vi "cameraControl.vi"(1 "Stream?":bool, 2 "Camera Parameters":T3 {"Pixel Format" items=["PIXEL_FORMAT_MONO8", "PIXEL_FORMAT_MONO16", "PIXEL_FORMAT_YUV422", "PIXEL_FORMAT_BAYER8_GRBG", "PIXEL_FORMAT_BAYER16_GRBG", "PIXEL_FORMAT_RGB24", "PIXEL_FORMAT_RGB48", "PIXEL_FORMAT_BAYER8_RGGB", "PIXEL_FORMAT_BAYER8_GBRG ", "PIXEL_FORMAT_BAYER8_BGGR ", "PIXEL_FORMAT_BAYER16_RGGB ", "PIXEL_FORMAT_BAYER16_GBRG", "PIXEL_FORMAT_BAYER16_BGGR", "PIXEL_FORMAT_RGB32"]}, 3 "Selector":u16(ring)) -> (0 "Camera Device OUT":T1)   [LabVIEW 2010]
uses:
  <vilib>/addons/PixeLINK/Low Level Functions/CAMERA_FEATURES.llb/TDPU-CameraFeatures-FeatureIds.ctl
  <vilib>/addons/PixeLINK/Low Level Functions/CAMERA_FEATURES.llb/TDPU-CameraFeatures-FeatureFlags.ctl
  <vilib>/addons/PixeLINK/Low Level Functions/CAMERA_FEATURES.llb/TDPU-CameraFeatures-PixelFormat.ctl
panel:
  in  "Camera Device IN":T1
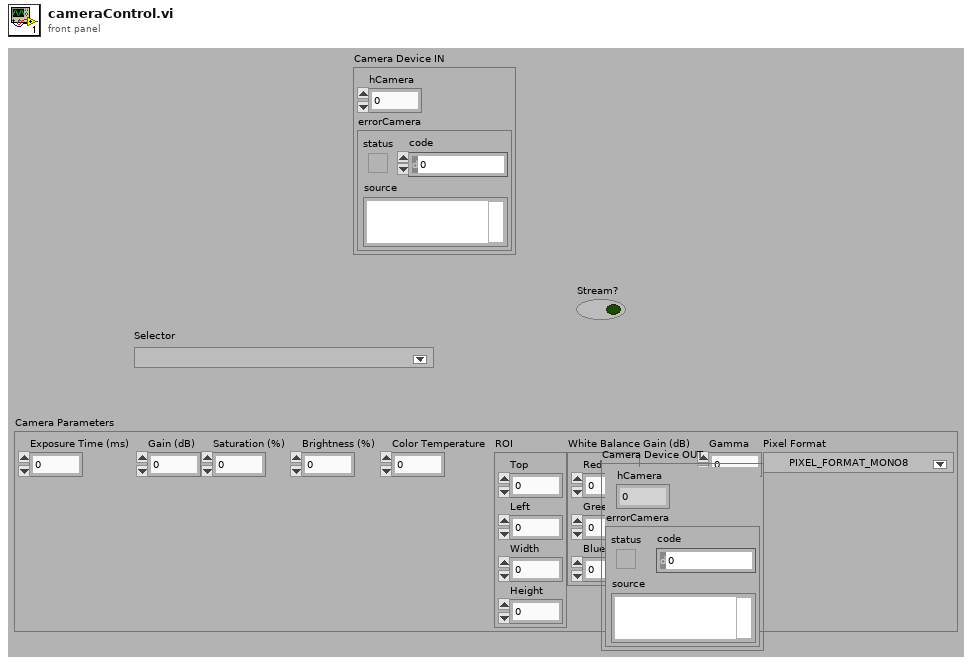
[diagram p1: front panel]
types:
  T1 = cluster{"hCamera":u32, "errorCamera":errorcluster}
  T2 = typedef "TDPU-CameraFeatures-PixelFormat.ctl" = u16
  T3 = cluster{"Exposure Time (ms)":dbl, "Gain (dB)":dbl, "Saturation (%)":dbl, "Brightness (%)":dbl, "Color Temperature":dbl, "ROI":cluster{"Top":i32, "Left":i32, "Width":i32, "Height":i32}, "White Balance Gain (dB)":cluster{"Red":dbl, "Green":dbl, "Blue":dbl}, "Gamma":dbl, "Pixel Format":T2}
  T4 = cluster{"Selector":u16, "Stream?":bool, "Camera Parameters":cluster{"Exposure Time (ms)":dbl, "Gain (dB)":dbl, "Saturation (%)":dbl, "Brightness (%)":dbl, "Color Temperature":dbl, "ROI":cluster{"Top":i32, "Left":i32, "Width":i32, "Height":i32}, "White Balance Gain (dB)":cluster{"Red":dbl, "Green":dbl, "Blue":dbl}, "Gamma":dbl, "Pixel Format":T2}}
  T5 = typedef "TDPU-CameraFeatures-FeatureFlags.ctl" = u32
  T6 = typedef "TDPU-CameraFeatures-FeatureIds.ctl" = u32
  T7 = cluster{"Top":i32, "Left":i32, "Width":i32, "Height":i32}
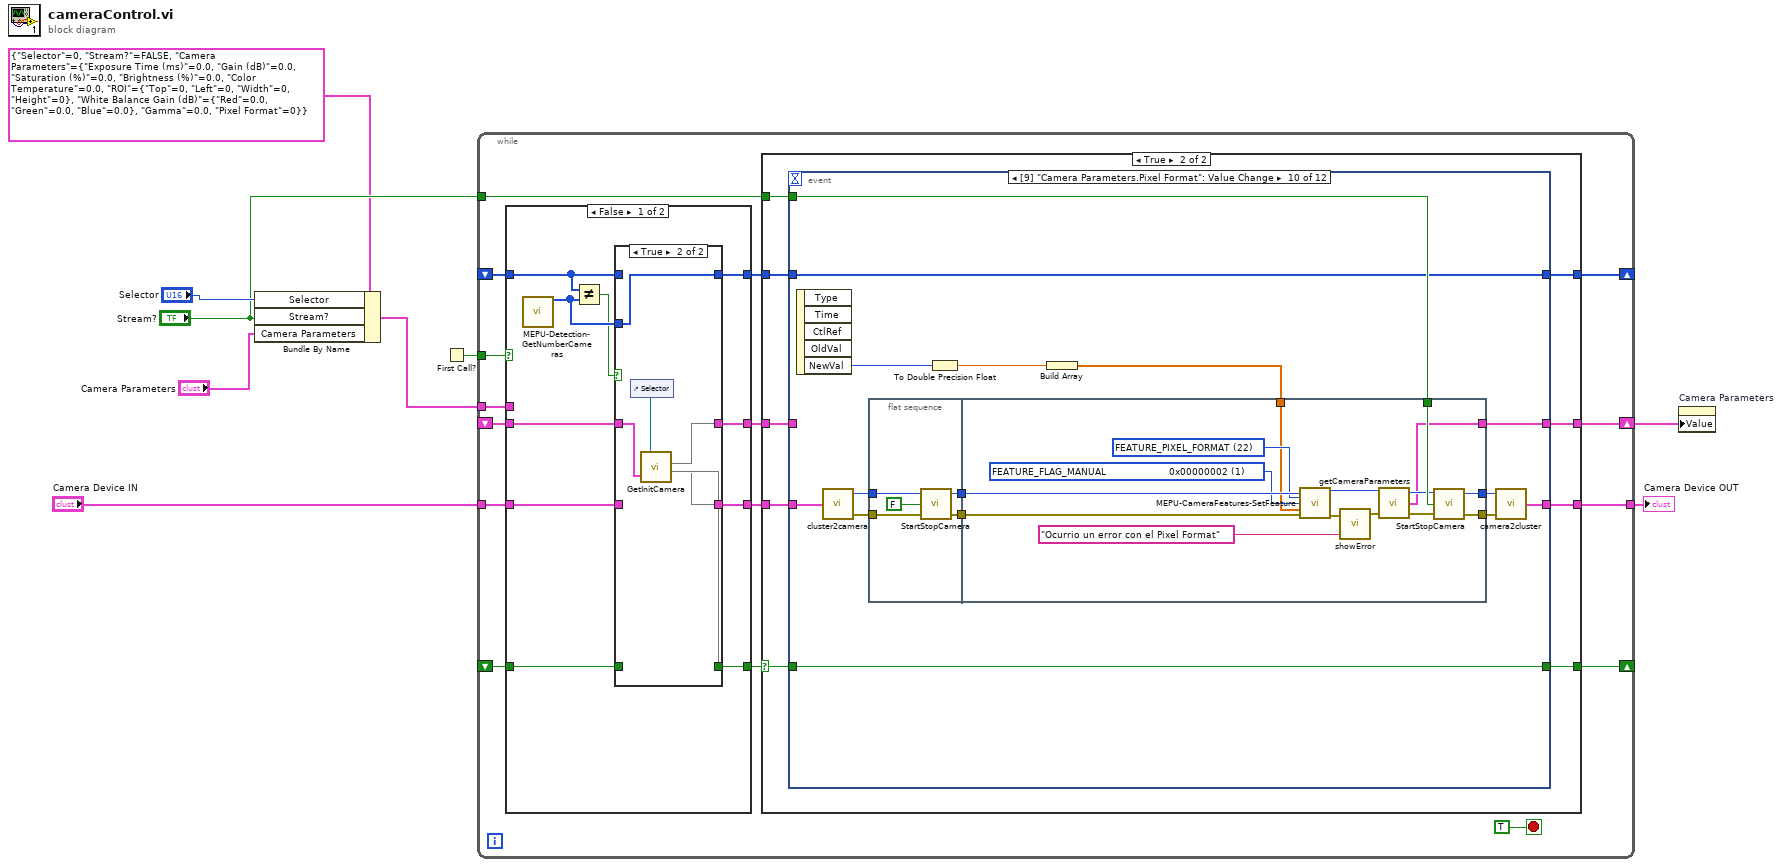
[diagram p0: block diagram]
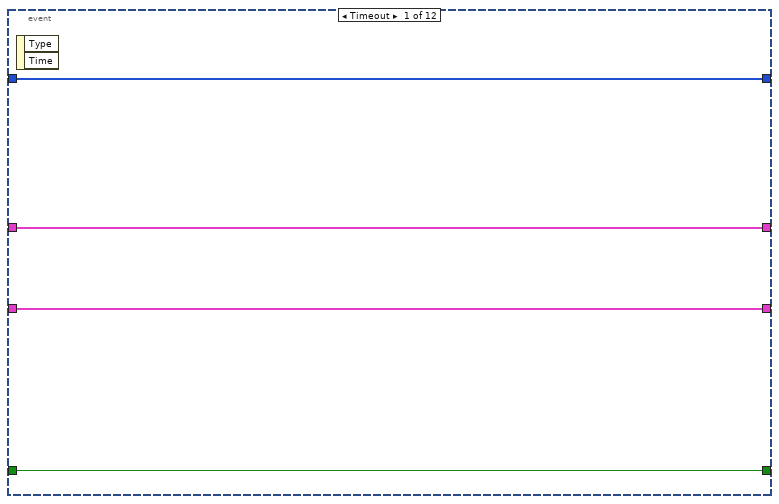
[diagram p3: hidden frame]
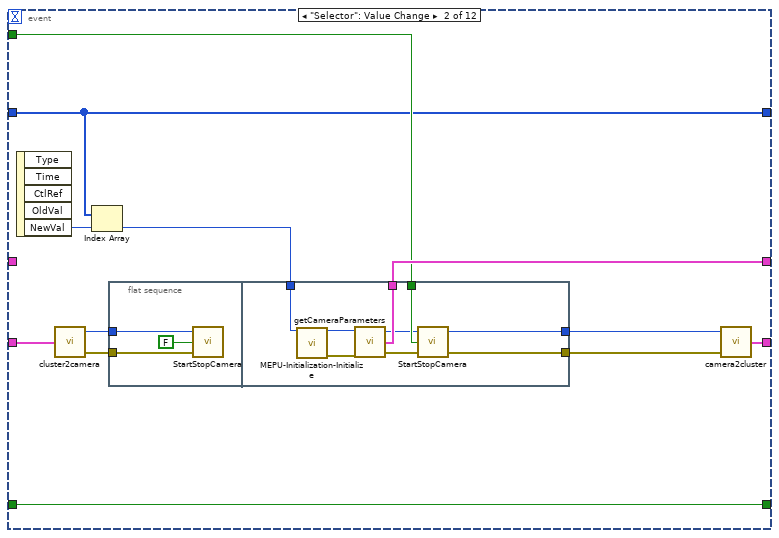
[diagram p4: hidden frame]
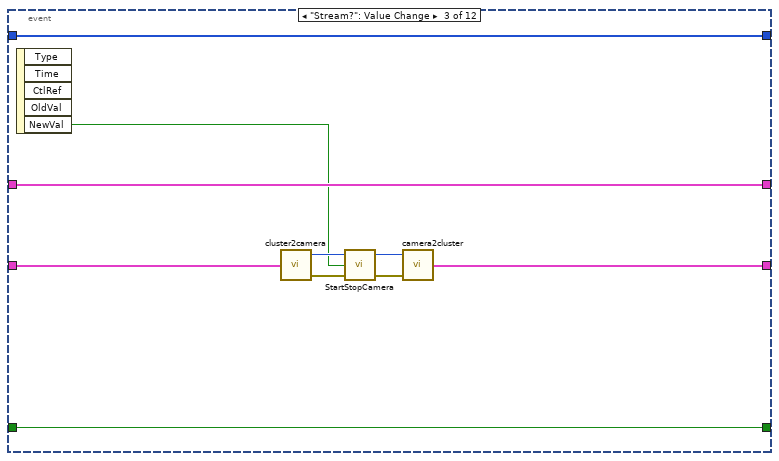
[diagram p5: hidden frame]
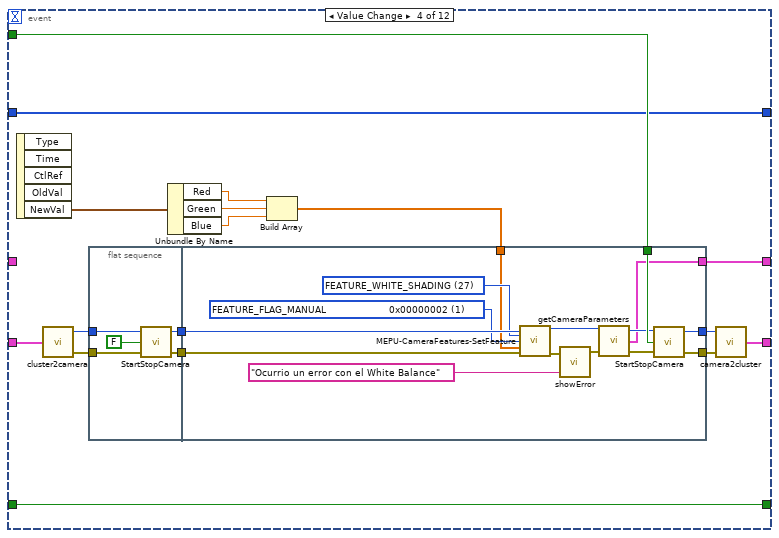
[diagram p6: hidden frame]
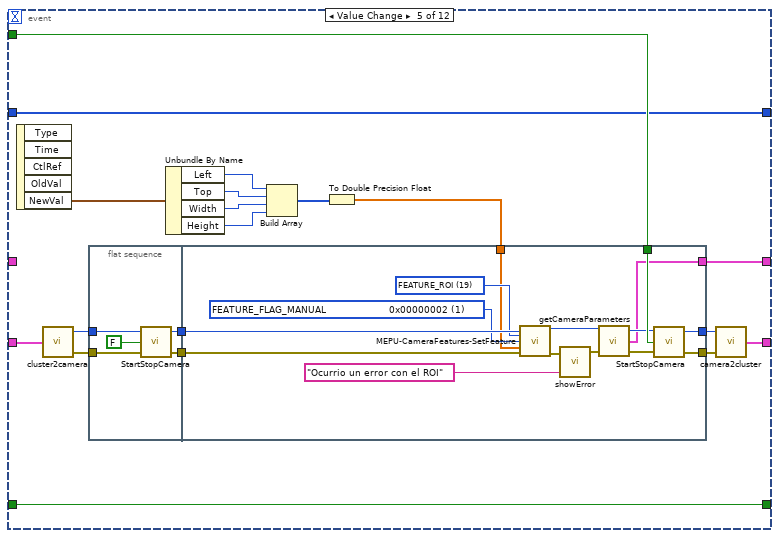
[diagram p7: hidden frame]
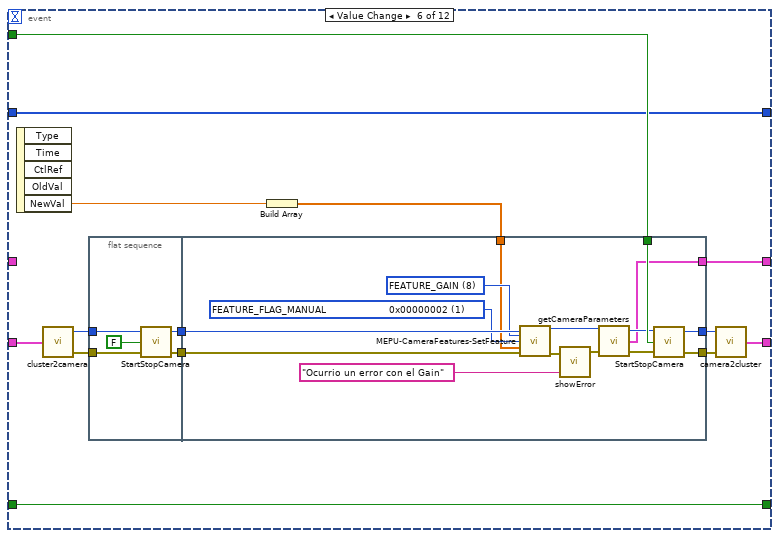
[diagram p8: hidden frame]
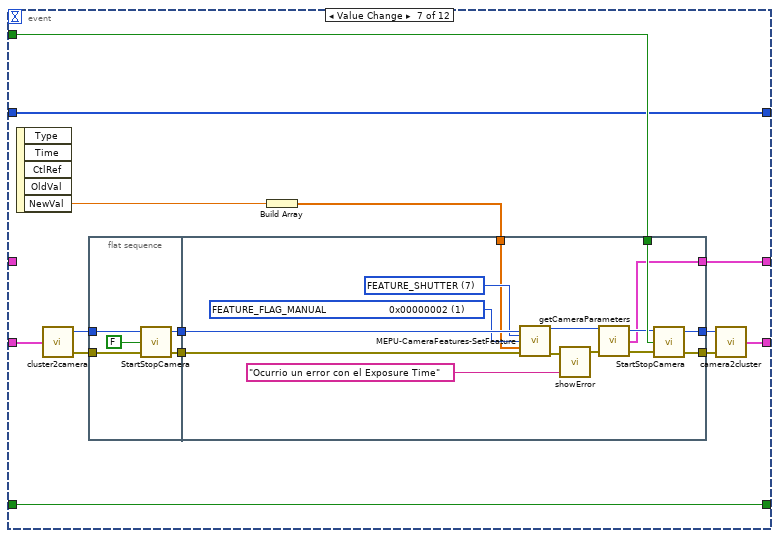
[diagram p9: hidden frame]
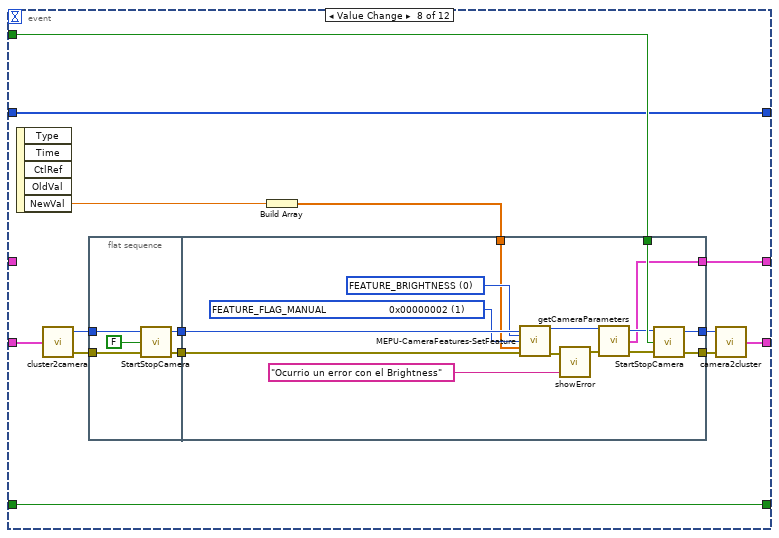
[diagram p10: hidden frame]
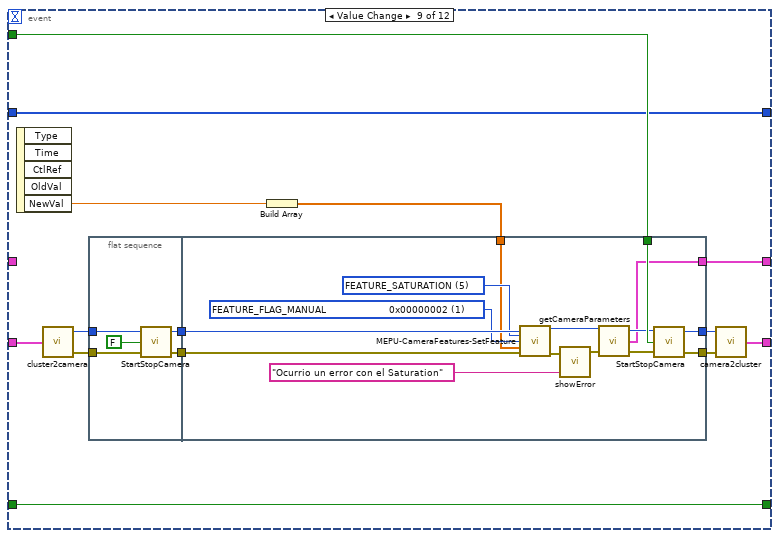
[diagram p11: hidden frame]
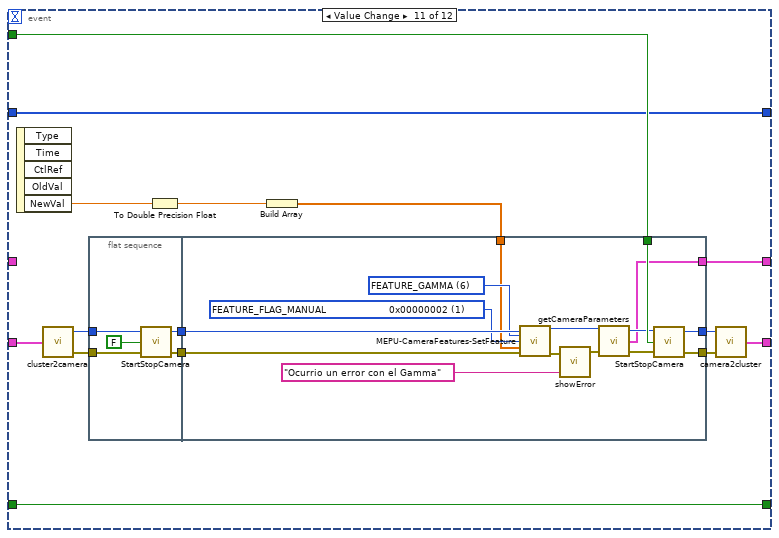
[diagram p12: hidden frame]
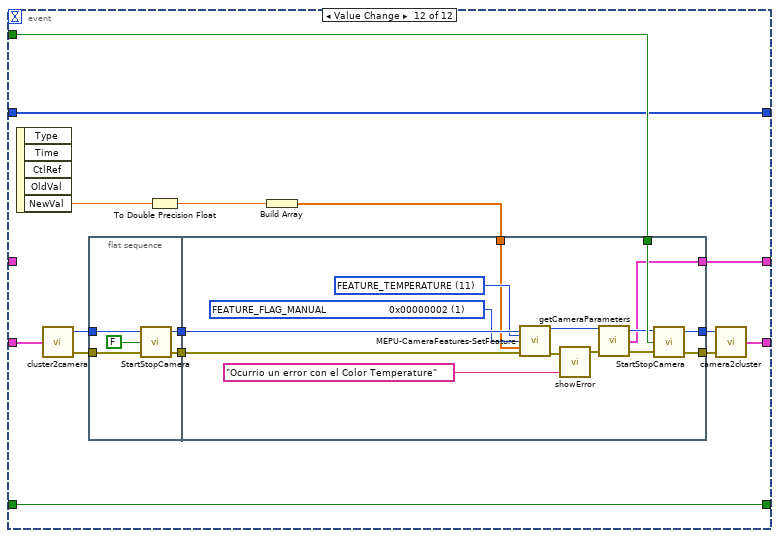
[diagram p13: hidden frame]
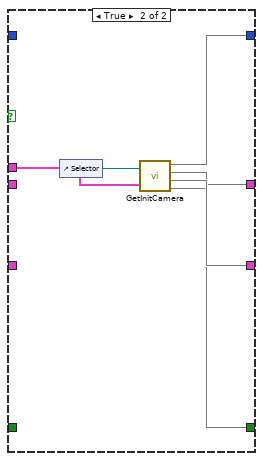
[diagram p15: hidden frame]
diagram:
  n1 = Bundle By Name(cluster=T4 {"Selector"=0, "Stream?"=FALSE, "Camera Parameters"={"Exposure Time (ms)"=0.0, "Gain (dB)"=0.0, "Saturation (%)"=0.0, "Brightness (%)"=0.0, "Color Temperature"=0.0, "ROI"={"Top"=0, "Left"=0, "Width"=0, "Height"=0}, "White Balance Gain (dB)"={"Red"=0.0, "Green"=0.0, "Blue"=0.0}, "Gamma"=0.0, "Pixel Format"=0}}, "Selector"="Selector", "Stream?"="Stream?", "Camera Parameters"="Camera Parameters") -> (w1:T4)
  n2 = First Call?() -> (First Call?: T/F=w9:bool)
  n3 = while {
    shift-right: [w23] -> w8
    shift-left: _ -> [w13]
    tunnel: "Stream?" -> [w22]
    tunnel: w9 -> [w19]
    shift-right: [w21] -> _
    shift-left: _ -> [w20]
    shift-right: [w18] -> _
    shift-left: _ -> [w12]
    tunnel: w1 -> [w11]
    tunnel: "Camera Device IN" -> [w15]
    tunnel: [w10] -> w7
    stop <- TRUE stop-if-true
    n4 = case shown="False" w19 {
      tunnel: [w400 w419] -> w24
      tunnel: w20 -> [w399 _]
      tunnel: [w402 w418] -> w17
      tunnel: [w403 w417] -> w16
      tunnel: w15 -> [w396 _]
      tunnel: [w401 w416] -> w14
      tunnel: w13 -> [w397 _]
      tunnel: w12 -> [w395 _]
      tunnel: w11 -> [_ w415]
      frame False {
        n5 = call <vilib>:"MEPU-Detection-GetNumberCameras.vi"() -> ("LV_SerialNumbers OUT"=w398:u32[])  [unwired: 13 in, 2 out]
        n6 = Not Equal?(x=w399, y=w398) -> (x != y?=w394:bool)
        n7 = case shown="True" w394 {
          tunnel: [w404 w413] -> w403
          tunnel: [w405 w412] -> w402
          tunnel: [w406 w411] -> w401
          tunnel: [w407 w408] -> w400
          tunnel: w399 -> [w407 _]
          tunnel: w398 -> [_ w408]
          tunnel: w397 -> [w406 w409]
          tunnel: w396 -> [w405 _]
          tunnel: w395 -> [w404 _]
          frame False {
          }
          frame True {
            n8 = control-ref of="Selector"() -> (w410:refnum<vi>)
            n9 = call "GetInitCamera.vi"(0:w409, 1:w410) -> (2:w413, 3:w412, 4:w411)  [unwired: 1 in]
          }
        }
      }
      frame True {
        n10 = control-ref of="Selector"() -> (w414:refnum<vi>)
        n11 = call "GetInitCamera.vi"(0:w415, 1:w414) -> (2:w417, 3:w418, 4:w416, 5:w419)
      }
    }
    n12 = case shown="True" w16 {
      selector: w16 -> [w26 w32]
      tunnel: w24 -> [w29 w38]
      tunnel: [w28 w37] -> w23
      tunnel: [w27 w36] -> w10
      tunnel: w22 -> [_ w35]
      tunnel: [w29 w34] -> w21
      tunnel: [w26 w33] -> w18
      tunnel: w17 -> [w27 w31]
      tunnel: w14 -> [w28 w30]
      frame False {
      }
      frame True {
        n13 = event shown="[9] \"Camera Parameters.Pixel Format\": Value Change" {
          selector: _ -> [_ _ _ _ _ _ _ _ _ _ _ _]
          dyn-events: _ -> [_ _ _ _ _ _ _ _ _ _ _ _]
          timeout: _ -> [_ _ _ _ _ _ _ _ _ _ _ _]
          tunnel: w38 -> [w40 w44 w69 w78 w117 w154 w188 w222 w256 w292 w327 w362]
          tunnel: [w42 w48 w70 w83 w122 w157 w191 w225 w259 w294 w329 w364] -> w37
          tunnel: [w41 w53 w75 w88 w127 w161 w195 w229 w263 w298 w333 w368] -> w36
          tunnel: w35 -> [_ w47 _ w85 w124 w158 w192 w226 w260 w295 w330 w365]
          tunnel: w30 -> [w42 _ w70 _ _ _ _ _ _ _ _ _]
          tunnel: w31 -> [w41 w52 w76 w89 w128 w162 w196 w230 w264 w299 w334 w369]
          tunnel: [w40 w44 w69 w78 w117 w154 w188 w222 w256 w292 w327 w362] -> w34
          tunnel: [w39 w43 w67 w77 w114 w153 w187 w221 w255 w289 w324 w359] -> w33
          tunnel: w32 -> [w39 w43 w67 w77 w114 w153 w187 w221 w255 w289 w324 w359]
          event Timeout {
            n14 = event-data() -> ()  [unwired: 1 in, 2 out]
          }
          event "Selector": Value Change {
            n15 = event-data() -> ("NewVal"=w54:u16)  [unwired: 1 in, 4 out]
            n16 = call "cluster2camera.vi"("Camera Device IN"=w52) -> ("Error OUT"=w50:errorcluster, "hCamera OUT"=w51:u32)  [unwired: 1 in]
            n17 = Index Array(array=w44, index=w54) -> (element=w49:u32)
            n18 = flat-sequence {
              tunnel: w51 -> [w56]
              tunnel: w50 -> [w55]
              tunnel: w49 -> [w66]
              tunnel: [w62] -> w48
              tunnel: w47 -> [w61]
              tunnel: [w59] -> w46
              tunnel: [w58] -> w45
              frame #0 {
                n19 = call "StartStopCamera.vi"("Error IN"=w55, "Camara ON?"=FALSE, "hCamera IN"=w56) -> ()  [unwired: 1 in, 2 out]
              }
              frame #1 {
                n20 = call <vilib>:"MEPU-Initialization-Initialize.vi"("uSerialNumber IN"=w66) -> ("phCamera OUT"=w65:u32, "Error OUT"=w64:errorcluster)  [unwired: 12 in, 1 out]
                n21 = call "getCameraParameters.vi"("Error IN"=w64, "hCamera IN"=w65) -> ("Error OUT"=w63:errorcluster, "Camera Parameters"=w62:T3, "hCamera OUT"=w60:u32)  [unwired: 1 in]
                n22 = call "StartStopCamera.vi"("Error IN"=w63, "Camara ON?"=w61, "hCamera IN"=w60) -> ("Error OUT"=w58:errorcluster, "hCamera OUT"=w59:u32)  [unwired: 1 in]
              }
            }
            n23 = call "camera2cluster.vi"("Error IN"=w45, "hCamera IN"=w46) -> ("Camera Device OUT"=w53:T1)  [unwired: 1 in]
          }
          event "Stream?": Value Change {
            n24 = event-data() -> ("NewVal"=w68:bool)  [unwired: 1 in, 4 out]
            n25 = call "cluster2camera.vi"("Camera Device IN"=w76) -> ("Error OUT"=w73:errorcluster, "hCamera OUT"=w74:u32)  [unwired: 1 in]
            n26 = call "StartStopCamera.vi"("Error IN"=w73, "Camara ON?"=w68, "hCamera IN"=w74) -> ("Error OUT"=w71:errorcluster, "hCamera OUT"=w72:u32)  [unwired: 1 in]
            n27 = call "camera2cluster.vi"("Error IN"=w71, "hCamera IN"=w72) -> ("Camera Device OUT"=w75:T1)  [unwired: 1 in]
          }
          event "Camera Parameters.White Balance Gain (dB)": Value Change {
            n28 = event-data() -> ("NewVal"=w84:cluster{"Red":dbl, "Green":dbl, "Blue":dbl})  [unwired: 1 in, 4 out]
            n29 = call "cluster2camera.vi"("Camera Device IN"=w89) -> ("Error OUT"=w92:errorcluster, "hCamera OUT"=w93:u32)  [unwired: 1 in]
            n30 = flat-sequence {
              tunnel: w93 -> [w97]
              tunnel: w92 -> [w96]
              tunnel: [w95] -> w87
              tunnel: [w94] -> w86
              tunnel: w85 -> [w113]
              tunnel: [w112] -> w91
              tunnel: [w111] -> w90
              tunnel: w87 -> [w110]
              tunnel: w86 -> [w109]
              tunnel: [w103] -> w83
              tunnel: w79 -> [w102]
              frame #0 {
                n31 = call "StartStopCamera.vi"("Error IN"=w96, "Camara ON?"=FALSE, "hCamera IN"=w97) -> ("Error OUT"=w94:errorcluster, "hCamera OUT"=w95:u32)  [unwired: 1 in]
              }
              frame #1 {
                w107 = T5 1 items=["FEATURE_FLAG_PRESENCE                 0x00000001", "FEATURE_FLAG_MANUAL                     0x00000002", "FEATURE_FLAG_AUTO                         0x00000004", "FEATURE_FLAG_ONEPUSH                   0x00000008", "FEATURE_FLAG_OFF                            0x00000010", "FEATURE_FLAG_DESC_SUPPORTED    0x00000020", "FEATURE_FLAG_READ_ONLY               0x00000040"] ("uFlags IN")
                w108 = T6 27 items=["FEATURE_BRIGHTNESS", "FEATURE_EXPOSURE", "FEATURE_SHARPNESS", "FEATURE_WHITE_BAL", "FEATURE_HUE", "FEATURE_SATURATION", "FEATURE_GAMMA", "FEATURE_SHUTTER", "FEATURE_GAIN", "FEATURE_IRIS", "FEATURE_FOCUS", "FEATURE_TEMPERATURE", "FEATURE_TRIGGER", "FEATURE_ZOOM", "FEATURE_PAN", "FEATURE_TILT", "FEATURE_OPT_FILTER", "FEATURE_GPIO", "FEATURE_FRAME_RATE", "FEATURE_ROI", "FEATURE_FLIP", "FEATURE_PIXEL_ADDRESSING", "FEATURE_PIXEL_FORMAT", "FEATURE_EXTENDED_SHUTTER", "FEATURE_AUTO_ROI", "FEATURE_LOOKUP_TABLE", "FEATURE_MEMORY_CHANNEL", "FEATURE_WHITE_SHADING", "FEATURE_ROTATE", "FEATURE_IMAGER_CLK_DIVISOR", "FEATURE_TRIG_WITH_CNTRLD_LIGHT", "FEATURE_MAX_PIXEL_SIZE"] ("uFeatureId IN")
                n32 = call <vilib>:"MEPU-CameraFeatures-SetFeature.vi"("hCamera IN"=w110, "uFeatureId IN"=w108, "uFlags IN"=w107, "pParms IN"=w102, "Error IN"=w109) -> ("hCamera OUT"=w106:u32, "Error OUT"=w101:errorcluster)  [unwired: 8 in, 1 out]
                n33 = call "showError.vi"("message"="Ocurrio un error con el White Balance", "Error IN"=w101) -> ("Error OUT"=w100:errorcluster)  [unwired: 3 in]
                n34 = call "getCameraParameters.vi"("Error IN"=w100, "hCamera IN"=w106) -> ("Error OUT"=w104:errorcluster, "Camera Parameters"=w103:T3, "hCamera OUT"=w105:u32)  [unwired: 1 in]
                n35 = call "StartStopCamera.vi"("Error IN"=w104, "Camara ON?"=w113, "hCamera IN"=w105) -> ("Error OUT"=w111:errorcluster, "hCamera OUT"=w112:u32)  [unwired: 1 in]
              }
            }
            n36 = Unbundle By Name(w84) -> ("Red"=w82:dbl, "Green"=w81:dbl, "Blue"=w80:dbl)
            n37 = Build Array(w82, w81, w80) -> (w79:dbl[])
            n38 = call "camera2cluster.vi"("Error IN"=w90, "hCamera IN"=w91) -> ("Camera Device OUT"=w88:T1)  [unwired: 1 in]
          }
          event "Camera Parameters.ROI": Value Change {
            n39 = event-data() -> ("NewVal"=w123:T7)  [unwired: 1 in, 4 out]
            n40 = call "cluster2camera.vi"("Camera Device IN"=w128) -> ("Error OUT"=w131:errorcluster, "hCamera OUT"=w132:u32)  [unwired: 1 in]
            n41 = flat-sequence {
              tunnel: w132 -> [w136]
              tunnel: w131 -> [w135]
              tunnel: [w134] -> w126
              tunnel: [w133] -> w125
              tunnel: w124 -> [w152]
              tunnel: [w151] -> w130
              tunnel: [w150] -> w129
              tunnel: w126 -> [w149]
              tunnel: w125 -> [w148]
              tunnel: [w142] -> w122
              tunnel: w115 -> [w141]
              frame #0 {
                n42 = call "StartStopCamera.vi"("Error IN"=w135, "Camara ON?"=FALSE, "hCamera IN"=w136) -> ("Error OUT"=w133:errorcluster, "hCamera OUT"=w134:u32)  [unwired: 1 in]
              }
              frame #1 {
                w146 = T5 1 items=["FEATURE_FLAG_PRESENCE                 0x00000001", "FEATURE_FLAG_MANUAL                     0x00000002", "FEATURE_FLAG_AUTO                         0x00000004", "FEATURE_FLAG_ONEPUSH                   0x00000008", "FEATURE_FLAG_OFF                            0x00000010", "FEATURE_FLAG_DESC_SUPPORTED    0x00000020", "FEATURE_FLAG_READ_ONLY               0x00000040"] ("uFlags IN")
                w147 = T6 19 items=["FEATURE_BRIGHTNESS", "FEATURE_EXPOSURE", "FEATURE_SHARPNESS", "FEATURE_WHITE_BAL", "FEATURE_HUE", "FEATURE_SATURATION", "FEATURE_GAMMA", "FEATURE_SHUTTER", "FEATURE_GAIN", "FEATURE_IRIS", "FEATURE_FOCUS", "FEATURE_TEMPERATURE", "FEATURE_TRIGGER", "FEATURE_ZOOM", "FEATURE_PAN", "FEATURE_TILT", "FEATURE_OPT_FILTER", "FEATURE_GPIO", "FEATURE_FRAME_RATE", "FEATURE_ROI", "FEATURE_FLIP", "FEATURE_PIXEL_ADDRESSING", "FEATURE_PIXEL_FORMAT", "FEATURE_EXTENDED_SHUTTER", "FEATURE_AUTO_ROI", "FEATURE_LOOKUP_TABLE", "FEATURE_MEMORY_CHANNEL", "FEATURE_WHITE_SHADING", "FEATURE_ROTATE", "FEATURE_IMAGER_CLK_DIVISOR", "FEATURE_TRIG_WITH_CNTRLD_LIGHT", "FEATURE_MAX_PIXEL_SIZE"] ("uFeatureId IN")
                n43 = call <vilib>:"MEPU-CameraFeatures-SetFeature.vi"("hCamera IN"=w149, "uFeatureId IN"=w147, "uFlags IN"=w146, "pParms IN"=w141, "Error IN"=w148) -> ("hCamera OUT"=w145:u32, "Error OUT"=w140:errorcluster)  [unwired: 8 in, 1 out]
                n44 = call "showError.vi"("message"="Ocurrio un error con el ROI", "Error IN"=w140) -> ("Error OUT"=w139:errorcluster)  [unwired: 3 in]
                n45 = call "getCameraParameters.vi"("Error IN"=w139, "hCamera IN"=w145) -> ("Error OUT"=w143:errorcluster, "Camera Parameters"=w142:T3, "hCamera OUT"=w144:u32)  [unwired: 1 in]
                n46 = call "StartStopCamera.vi"("Error IN"=w143, "Camara ON?"=w152, "hCamera IN"=w144) -> ("Error OUT"=w150:errorcluster, "hCamera OUT"=w151:u32)  [unwired: 1 in]
              }
            }
            n47 = Unbundle By Name(w123) -> ("Left"=w121:i32, "Top"=w120:i32, "Width"=w119:i32, "Height"=w118:i32)
            n48 = Build Array(w121, w120, w119, w118) -> (w116:i32[])
            n49 = To Double Precision Float(number=w116) -> (double precision float=w115:dbl[])
            n50 = call "camera2cluster.vi"("Error IN"=w129, "hCamera IN"=w130) -> ("Camera Device OUT"=w127:T1)  [unwired: 1 in]
          }
          event "Camera Parameters.Gain (dB)": Value Change {
            n51 = event-data() -> ("NewVal"=w155:dbl)  [unwired: 1 in, 4 out]
            n52 = call "cluster2camera.vi"("Camera Device IN"=w162) -> ("Error OUT"=w165:errorcluster, "hCamera OUT"=w166:u32)  [unwired: 1 in]
            n53 = flat-sequence {
              tunnel: w166 -> [w170]
              tunnel: w165 -> [w169]
              tunnel: [w168] -> w160
              tunnel: [w167] -> w159
              tunnel: w158 -> [w186]
              tunnel: [w185] -> w164
              tunnel: [w184] -> w163
              tunnel: w160 -> [w183]
              tunnel: w159 -> [w182]
              tunnel: [w176] -> w157
              tunnel: w156 -> [w175]
              frame #0 {
                n54 = call "StartStopCamera.vi"("Error IN"=w169, "Camara ON?"=FALSE, "hCamera IN"=w170) -> ("Error OUT"=w167:errorcluster, "hCamera OUT"=w168:u32)  [unwired: 1 in]
              }
              frame #1 {
                w180 = T5 1 items=["FEATURE_FLAG_PRESENCE                 0x00000001", "FEATURE_FLAG_MANUAL                     0x00000002", "FEATURE_FLAG_AUTO                         0x00000004", "FEATURE_FLAG_ONEPUSH                   0x00000008", "FEATURE_FLAG_OFF                            0x00000010", "FEATURE_FLAG_DESC_SUPPORTED    0x00000020", "FEATURE_FLAG_READ_ONLY               0x00000040"] ("uFlags IN")
                w181 = T6 8 items=["FEATURE_BRIGHTNESS", "FEATURE_EXPOSURE", "FEATURE_SHARPNESS", "FEATURE_WHITE_BAL", "FEATURE_HUE", "FEATURE_SATURATION", "FEATURE_GAMMA", "FEATURE_SHUTTER", "FEATURE_GAIN", "FEATURE_IRIS", "FEATURE_FOCUS", "FEATURE_TEMPERATURE", "FEATURE_TRIGGER", "FEATURE_ZOOM", "FEATURE_PAN", "FEATURE_TILT", "FEATURE_OPT_FILTER", "FEATURE_GPIO", "FEATURE_FRAME_RATE", "FEATURE_ROI", "FEATURE_FLIP", "FEATURE_PIXEL_ADDRESSING", "FEATURE_PIXEL_FORMAT", "FEATURE_EXTENDED_SHUTTER", "FEATURE_AUTO_ROI", "FEATURE_LOOKUP_TABLE", "FEATURE_MEMORY_CHANNEL", "FEATURE_WHITE_SHADING", "FEATURE_ROTATE", "FEATURE_IMAGER_CLK_DIVISOR", "FEATURE_TRIG_WITH_CNTRLD_LIGHT", "FEATURE_MAX_PIXEL_SIZE"] ("uFeatureId IN")
                n55 = call <vilib>:"MEPU-CameraFeatures-SetFeature.vi"("hCamera IN"=w183, "uFeatureId IN"=w181, "uFlags IN"=w180, "pParms IN"=w175, "Error IN"=w182) -> ("hCamera OUT"=w179:u32, "Error OUT"=w174:errorcluster)  [unwired: 8 in, 1 out]
                n56 = call "showError.vi"("message"="Ocurrio un error con el Gain", "Error IN"=w174) -> ("Error OUT"=w173:errorcluster)  [unwired: 3 in]
                n57 = call "getCameraParameters.vi"("Error IN"=w173, "hCamera IN"=w179) -> ("Error OUT"=w177:errorcluster, "Camera Parameters"=w176:T3, "hCamera OUT"=w178:u32)  [unwired: 1 in]
                n58 = call "StartStopCamera.vi"("Error IN"=w177, "Camara ON?"=w186, "hCamera IN"=w178) -> ("Error OUT"=w184:errorcluster, "hCamera OUT"=w185:u32)  [unwired: 1 in]
              }
            }
            n59 = Build Array(w155) -> (w156:dbl[])
            n60 = call "camera2cluster.vi"("Error IN"=w163, "hCamera IN"=w164) -> ("Camera Device OUT"=w161:T1)  [unwired: 1 in]
          }
          event "Camera Parameters.Exposure Time (ms)": Value Change {
            n61 = event-data() -> ("NewVal"=w189:dbl)  [unwired: 1 in, 4 out]
            n62 = call "cluster2camera.vi"("Camera Device IN"=w196) -> ("Error OUT"=w199:errorcluster, "hCamera OUT"=w200:u32)  [unwired: 1 in]
            n63 = flat-sequence {
              tunnel: w200 -> [w204]
              tunnel: w199 -> [w203]
              tunnel: [w202] -> w194
              tunnel: [w201] -> w193
              tunnel: w192 -> [w220]
              tunnel: [w219] -> w198
              tunnel: [w218] -> w197
              tunnel: w194 -> [w217]
              tunnel: w193 -> [w216]
              tunnel: [w210] -> w191
              tunnel: w190 -> [w209]
              frame #0 {
                n64 = call "StartStopCamera.vi"("Error IN"=w203, "Camara ON?"=FALSE, "hCamera IN"=w204) -> ("Error OUT"=w201:errorcluster, "hCamera OUT"=w202:u32)  [unwired: 1 in]
              }
              frame #1 {
                w214 = T5 1 items=["FEATURE_FLAG_PRESENCE                 0x00000001", "FEATURE_FLAG_MANUAL                     0x00000002", "FEATURE_FLAG_AUTO                         0x00000004", "FEATURE_FLAG_ONEPUSH                   0x00000008", "FEATURE_FLAG_OFF                            0x00000010", "FEATURE_FLAG_DESC_SUPPORTED    0x00000020", "FEATURE_FLAG_READ_ONLY               0x00000040"] ("uFlags IN")
                w215 = T6 7 items=["FEATURE_BRIGHTNESS", "FEATURE_EXPOSURE", "FEATURE_SHARPNESS", "FEATURE_WHITE_BAL", "FEATURE_HUE", "FEATURE_SATURATION", "FEATURE_GAMMA", "FEATURE_SHUTTER", "FEATURE_GAIN", "FEATURE_IRIS", "FEATURE_FOCUS", "FEATURE_TEMPERATURE", "FEATURE_TRIGGER", "FEATURE_ZOOM", "FEATURE_PAN", "FEATURE_TILT", "FEATURE_OPT_FILTER", "FEATURE_GPIO", "FEATURE_FRAME_RATE", "FEATURE_ROI", "FEATURE_FLIP", "FEATURE_PIXEL_ADDRESSING", "FEATURE_PIXEL_FORMAT", "FEATURE_EXTENDED_SHUTTER", "FEATURE_AUTO_ROI", "FEATURE_LOOKUP_TABLE", "FEATURE_MEMORY_CHANNEL", "FEATURE_WHITE_SHADING", "FEATURE_ROTATE", "FEATURE_IMAGER_CLK_DIVISOR", "FEATURE_TRIG_WITH_CNTRLD_LIGHT", "FEATURE_MAX_PIXEL_SIZE"] ("uFeatureId IN")
                n65 = call <vilib>:"MEPU-CameraFeatures-SetFeature.vi"("hCamera IN"=w217, "uFeatureId IN"=w215, "uFlags IN"=w214, "pParms IN"=w209, "Error IN"=w216) -> ("hCamera OUT"=w213:u32, "Error OUT"=w208:errorcluster)  [unwired: 8 in, 1 out]
                n66 = call "showError.vi"("message"="Ocurrio un error con el Exposure Time", "Error IN"=w208) -> ("Error OUT"=w207:errorcluster)  [unwired: 3 in]
                n67 = call "getCameraParameters.vi"("Error IN"=w207, "hCamera IN"=w213) -> ("Error OUT"=w211:errorcluster, "Camera Parameters"=w210:T3, "hCamera OUT"=w212:u32)  [unwired: 1 in]
                n68 = call "StartStopCamera.vi"("Error IN"=w211, "Camara ON?"=w220, "hCamera IN"=w212) -> ("Error OUT"=w218:errorcluster, "hCamera OUT"=w219:u32)  [unwired: 1 in]
              }
            }
            n69 = Build Array(w189) -> (w190:dbl[])
            n70 = call "camera2cluster.vi"("Error IN"=w197, "hCamera IN"=w198) -> ("Camera Device OUT"=w195:T1)  [unwired: 1 in]
          }
          event "Camera Parameters.Brightness (%)": Value Change {
            n71 = event-data() -> ("NewVal"=w223:dbl)  [unwired: 1 in, 4 out]
            n72 = call "cluster2camera.vi"("Camera Device IN"=w230) -> ("Error OUT"=w233:errorcluster, "hCamera OUT"=w234:u32)  [unwired: 1 in]
            n73 = flat-sequence {
              tunnel: w234 -> [w238]
              tunnel: w233 -> [w237]
              tunnel: [w236] -> w228
              tunnel: [w235] -> w227
              tunnel: w226 -> [w254]
              tunnel: [w253] -> w232
              tunnel: [w252] -> w231
              tunnel: w228 -> [w251]
              tunnel: w227 -> [w250]
              tunnel: [w244] -> w225
              tunnel: w224 -> [w243]
              frame #0 {
                n74 = call "StartStopCamera.vi"("Error IN"=w237, "Camara ON?"=FALSE, "hCamera IN"=w238) -> ("Error OUT"=w235:errorcluster, "hCamera OUT"=w236:u32)  [unwired: 1 in]
              }
              frame #1 {
                w248 = T5 1 items=["FEATURE_FLAG_PRESENCE                 0x00000001", "FEATURE_FLAG_MANUAL                     0x00000002", "FEATURE_FLAG_AUTO                         0x00000004", "FEATURE_FLAG_ONEPUSH                   0x00000008", "FEATURE_FLAG_OFF                            0x00000010", "FEATURE_FLAG_DESC_SUPPORTED    0x00000020", "FEATURE_FLAG_READ_ONLY               0x00000040"] ("uFlags IN")
                w249 = T6 0 items=["FEATURE_BRIGHTNESS", "FEATURE_EXPOSURE", "FEATURE_SHARPNESS", "FEATURE_WHITE_BAL", "FEATURE_HUE", "FEATURE_SATURATION", "FEATURE_GAMMA", "FEATURE_SHUTTER", "FEATURE_GAIN", "FEATURE_IRIS", "FEATURE_FOCUS", "FEATURE_TEMPERATURE", "FEATURE_TRIGGER", "FEATURE_ZOOM", "FEATURE_PAN", "FEATURE_TILT", "FEATURE_OPT_FILTER", "FEATURE_GPIO", "FEATURE_FRAME_RATE", "FEATURE_ROI", "FEATURE_FLIP", "FEATURE_PIXEL_ADDRESSING", "FEATURE_PIXEL_FORMAT", "FEATURE_EXTENDED_SHUTTER", "FEATURE_AUTO_ROI", "FEATURE_LOOKUP_TABLE", "FEATURE_MEMORY_CHANNEL", "FEATURE_WHITE_SHADING", "FEATURE_ROTATE", "FEATURE_IMAGER_CLK_DIVISOR", "FEATURE_TRIG_WITH_CNTRLD_LIGHT", "FEATURE_MAX_PIXEL_SIZE"] ("uFeatureId IN")
                n75 = call <vilib>:"MEPU-CameraFeatures-SetFeature.vi"("hCamera IN"=w251, "uFeatureId IN"=w249, "uFlags IN"=w248, "pParms IN"=w243, "Error IN"=w250) -> ("hCamera OUT"=w247:u32, "Error OUT"=w242:errorcluster)  [unwired: 8 in, 1 out]
                n76 = call "showError.vi"("message"="Ocurrio un error con el Brightness", "Error IN"=w242) -> ("Error OUT"=w241:errorcluster)  [unwired: 3 in]
                n77 = call "getCameraParameters.vi"("Error IN"=w241, "hCamera IN"=w247) -> ("Error OUT"=w245:errorcluster, "Camera Parameters"=w244:T3, "hCamera OUT"=w246:u32)  [unwired: 1 in]
                n78 = call "StartStopCamera.vi"("Error IN"=w245, "Camara ON?"=w254, "hCamera IN"=w246) -> ("Error OUT"=w252:errorcluster, "hCamera OUT"=w253:u32)  [unwired: 1 in]
              }
            }
            n79 = Build Array(w223) -> (w224:dbl[])
            n80 = call "camera2cluster.vi"("Error IN"=w231, "hCamera IN"=w232) -> ("Camera Device OUT"=w229:T1)  [unwired: 1 in]
          }
          event "Camera Parameters.Saturation (%)": Value Change {
            n81 = event-data() -> ("NewVal"=w257:dbl)  [unwired: 1 in, 4 out]
            n82 = call "cluster2camera.vi"("Camera Device IN"=w264) -> ("Error OUT"=w267:errorcluster, "hCamera OUT"=w268:u32)  [unwired: 1 in]
            n83 = flat-sequence {
              tunnel: w268 -> [w272]
              tunnel: w267 -> [w271]
              tunnel: [w270] -> w262
              tunnel: [w269] -> w261
              tunnel: w260 -> [w288]
              tunnel: [w287] -> w266
              tunnel: [w286] -> w265
              tunnel: w262 -> [w285]
              tunnel: w261 -> [w284]
              tunnel: [w278] -> w259
              tunnel: w258 -> [w277]
              frame #0 {
                n84 = call "StartStopCamera.vi"("Error IN"=w271, "Camara ON?"=FALSE, "hCamera IN"=w272) -> ("Error OUT"=w269:errorcluster, "hCamera OUT"=w270:u32)  [unwired: 1 in]
              }
              frame #1 {
                w282 = T5 1 items=["FEATURE_FLAG_PRESENCE                 0x00000001", "FEATURE_FLAG_MANUAL                     0x00000002", "FEATURE_FLAG_AUTO                         0x00000004", "FEATURE_FLAG_ONEPUSH                   0x00000008", "FEATURE_FLAG_OFF                            0x00000010", "FEATURE_FLAG_DESC_SUPPORTED    0x00000020", "FEATURE_FLAG_READ_ONLY               0x00000040"] ("uFlags IN")
                w283 = T6 5 items=["FEATURE_BRIGHTNESS", "FEATURE_EXPOSURE", "FEATURE_SHARPNESS", "FEATURE_WHITE_BAL", "FEATURE_HUE", "FEATURE_SATURATION", "FEATURE_GAMMA", "FEATURE_SHUTTER", "FEATURE_GAIN", "FEATURE_IRIS", "FEATURE_FOCUS", "FEATURE_TEMPERATURE", "FEATURE_TRIGGER", "FEATURE_ZOOM", "FEATURE_PAN", "FEATURE_TILT", "FEATURE_OPT_FILTER", "FEATURE_GPIO", "FEATURE_FRAME_RATE", "FEATURE_ROI", "FEATURE_FLIP", "FEATURE_PIXEL_ADDRESSING", "FEATURE_PIXEL_FORMAT", "FEATURE_EXTENDED_SHUTTER", "FEATURE_AUTO_ROI", "FEATURE_LOOKUP_TABLE", "FEATURE_MEMORY_CHANNEL", "FEATURE_WHITE_SHADING", "FEATURE_ROTATE", "FEATURE_IMAGER_CLK_DIVISOR", "FEATURE_TRIG_WITH_CNTRLD_LIGHT", "FEATURE_MAX_PIXEL_SIZE"] ("uFeatureId IN")
                n85 = call <vilib>:"MEPU-CameraFeatures-SetFeature.vi"("hCamera IN"=w285, "uFeatureId IN"=w283, "uFlags IN"=w282, "pParms IN"=w277, "Error IN"=w284) -> ("hCamera OUT"=w281:u32, "Error OUT"=w276:errorcluster)  [unwired: 8 in, 1 out]
                n86 = call "showError.vi"("message"="Ocurrio un error con el Saturation", "Error IN"=w276) -> ("Error OUT"=w275:errorcluster)  [unwired: 3 in]
                n87 = call "getCameraParameters.vi"("Error IN"=w275, "hCamera IN"=w281) -> ("Error OUT"=w279:errorcluster, "Camera Parameters"=w278:T3, "hCamera OUT"=w280:u32)  [unwired: 1 in]
                n88 = call "StartStopCamera.vi"("Error IN"=w279, "Camara ON?"=w288, "hCamera IN"=w280) -> ("Error OUT"=w286:errorcluster, "hCamera OUT"=w287:u32)  [unwired: 1 in]
              }
            }
            n89 = Build Array(w257) -> (w258:dbl[])
            n90 = call "camera2cluster.vi"("Error IN"=w265, "hCamera IN"=w266) -> ("Camera Device OUT"=w263:T1)  [unwired: 1 in]
          }
          event Value Change {
            n91 = event-data() -> ("NewVal"=w291:T2)  [unwired: 1 in, 4 out]
            n92 = call "cluster2camera.vi"("Camera Device IN"=w299) -> ("Error OUT"=w302:errorcluster, "hCamera OUT"=w303:u32)  [unwired: 1 in]
            n93 = flat-sequence {
              tunnel: w303 -> [w307]
              tunnel: w302 -> [w306]
              tunnel: [w305] -> w297
              tunnel: [w304] -> w296
              tunnel: w295 -> [w323]
              tunnel: [w322] -> w301
              tunnel: [w321] -> w300
              tunnel: w297 -> [w320]
              tunnel: w296 -> [w319]
              tunnel: [w313] -> w294
              tunnel: w293 -> [w312]
              frame #0 {
                n94 = call "StartStopCamera.vi"("Error IN"=w306, "Camara ON?"=FALSE, "hCamera IN"=w307) -> ("Error OUT"=w304:errorcluster, "hCamera OUT"=w305:u32)  [unwired: 1 in]
              }
              frame #1 {
                w317 = T5 1 items=["FEATURE_FLAG_PRESENCE                 0x00000001", "FEATURE_FLAG_MANUAL                     0x00000002", "FEATURE_FLAG_AUTO                         0x00000004", "FEATURE_FLAG_ONEPUSH                   0x00000008", "FEATURE_FLAG_OFF                            0x00000010", "FEATURE_FLAG_DESC_SUPPORTED    0x00000020", "FEATURE_FLAG_READ_ONLY               0x00000040"] ("uFlags IN")
                w318 = T6 22 items=["FEATURE_BRIGHTNESS", "FEATURE_EXPOSURE", "FEATURE_SHARPNESS", "FEATURE_WHITE_BAL", "FEATURE_HUE", "FEATURE_SATURATION", "FEATURE_GAMMA", "FEATURE_SHUTTER", "FEATURE_GAIN", "FEATURE_IRIS", "FEATURE_FOCUS", "FEATURE_TEMPERATURE", "FEATURE_TRIGGER", "FEATURE_ZOOM", "FEATURE_PAN", "FEATURE_TILT", "FEATURE_OPT_FILTER", "FEATURE_GPIO", "FEATURE_FRAME_RATE", "FEATURE_ROI", "FEATURE_FLIP", "FEATURE_PIXEL_ADDRESSING", "FEATURE_PIXEL_FORMAT", "FEATURE_EXTENDED_SHUTTER", "FEATURE_AUTO_ROI", "FEATURE_LOOKUP_TABLE", "FEATURE_MEMORY_CHANNEL", "FEATURE_WHITE_SHADING", "FEATURE_ROTATE", "FEATURE_IMAGER_CLK_DIVISOR", "FEATURE_TRIG_WITH_CNTRLD_LIGHT", "FEATURE_MAX_PIXEL_SIZE"] ("uFeatureId IN")
                n95 = call <vilib>:"MEPU-CameraFeatures-SetFeature.vi"("hCamera IN"=w320, "uFeatureId IN"=w318, "uFlags IN"=w317, "pParms IN"=w312, "Error IN"=w319) -> ("hCamera OUT"=w316:u32, "Error OUT"=w311:errorcluster)  [unwired: 8 in, 1 out]
                n96 = call "showError.vi"("message"="Ocurrio un error con el Pixel Format", "Error IN"=w311) -> ("Error OUT"=w310:errorcluster)  [unwired: 3 in]
                n97 = call "getCameraParameters.vi"("Error IN"=w310, "hCamera IN"=w316) -> ("Error OUT"=w314:errorcluster, "Camera Parameters"=w313:T3, "hCamera OUT"=w315:u32)  [unwired: 1 in]
                n98 = call "StartStopCamera.vi"("Error IN"=w314, "Camara ON?"=w323, "hCamera IN"=w315) -> ("Error OUT"=w321:errorcluster, "hCamera OUT"=w322:u32)  [unwired: 1 in]
              }
            }
            n99 = To Double Precision Float(number=w291) -> (double precision float=w290:dbl)
            n100 = Build Array(w290) -> (w293:dbl[])
            n101 = call "camera2cluster.vi"("Error IN"=w300, "hCamera IN"=w301) -> ("Camera Device OUT"=w298:T1)  [unwired: 1 in]
          }
          event "Camera Parameters.Gamma": Value Change {
            n102 = event-data() -> ("NewVal"=w326:dbl)  [unwired: 1 in, 4 out]
            n103 = call "cluster2camera.vi"("Camera Device IN"=w334) -> ("Error OUT"=w337:errorcluster, "hCamera OUT"=w338:u32)  [unwired: 1 in]
            n104 = flat-sequence {
              tunnel: w338 -> [w342]
              tunnel: w337 -> [w341]
              tunnel: [w340] -> w332
              tunnel: [w339] -> w331
              tunnel: w330 -> [w358]
              tunnel: [w357] -> w336
              tunnel: [w356] -> w335
              tunnel: w332 -> [w355]
              tunnel: w331 -> [w354]
              tunnel: [w348] -> w329
              tunnel: w328 -> [w347]
              frame #0 {
                n105 = call "StartStopCamera.vi"("Error IN"=w341, "Camara ON?"=FALSE, "hCamera IN"=w342) -> ("Error OUT"=w339:errorcluster, "hCamera OUT"=w340:u32)  [unwired: 1 in]
              }
              frame #1 {
                w352 = T5 1 items=["FEATURE_FLAG_PRESENCE                 0x00000001", "FEATURE_FLAG_MANUAL                     0x00000002", "FEATURE_FLAG_AUTO                         0x00000004", "FEATURE_FLAG_ONEPUSH                   0x00000008", "FEATURE_FLAG_OFF                            0x00000010", "FEATURE_FLAG_DESC_SUPPORTED    0x00000020", "FEATURE_FLAG_READ_ONLY               0x00000040"] ("uFlags IN")
                w353 = T6 6 items=["FEATURE_BRIGHTNESS", "FEATURE_EXPOSURE", "FEATURE_SHARPNESS", "FEATURE_WHITE_BAL", "FEATURE_HUE", "FEATURE_SATURATION", "FEATURE_GAMMA", "FEATURE_SHUTTER", "FEATURE_GAIN", "FEATURE_IRIS", "FEATURE_FOCUS", "FEATURE_TEMPERATURE", "FEATURE_TRIGGER", "FEATURE_ZOOM", "FEATURE_PAN", "FEATURE_TILT", "FEATURE_OPT_FILTER", "FEATURE_GPIO", "FEATURE_FRAME_RATE", "FEATURE_ROI", "FEATURE_FLIP", "FEATURE_PIXEL_ADDRESSING", "FEATURE_PIXEL_FORMAT", "FEATURE_EXTENDED_SHUTTER", "FEATURE_AUTO_ROI", "FEATURE_LOOKUP_TABLE", "FEATURE_MEMORY_CHANNEL", "FEATURE_WHITE_SHADING", "FEATURE_ROTATE", "FEATURE_IMAGER_CLK_DIVISOR", "FEATURE_TRIG_WITH_CNTRLD_LIGHT", "FEATURE_MAX_PIXEL_SIZE"] ("uFeatureId IN")
                n106 = call <vilib>:"MEPU-CameraFeatures-SetFeature.vi"("hCamera IN"=w355, "uFeatureId IN"=w353, "uFlags IN"=w352, "pParms IN"=w347, "Error IN"=w354) -> ("hCamera OUT"=w351:u32, "Error OUT"=w346:errorcluster)  [unwired: 8 in, 1 out]
                n107 = call "showError.vi"("message"="Ocurrio un error con el Gamma", "Error IN"=w346) -> ("Error OUT"=w345:errorcluster)  [unwired: 3 in]
                n108 = call "getCameraParameters.vi"("Error IN"=w345, "hCamera IN"=w351) -> ("Error OUT"=w349:errorcluster, "Camera Parameters"=w348:T3, "hCamera OUT"=w350:u32)  [unwired: 1 in]
                n109 = call "StartStopCamera.vi"("Error IN"=w349, "Camara ON?"=w358, "hCamera IN"=w350) -> ("Error OUT"=w356:errorcluster, "hCamera OUT"=w357:u32)  [unwired: 1 in]
              }
            }
            n110 = To Double Precision Float(number=w326) -> (double precision float=w325:dbl)
            n111 = Build Array(w325) -> (w328:dbl[])
            n112 = call "camera2cluster.vi"("Error IN"=w335, "hCamera IN"=w336) -> ("Camera Device OUT"=w333:T1)  [unwired: 1 in]
          }
          event "Camera Parameters.Color Temperature": Value Change {
            n113 = event-data() -> ("NewVal"=w361:dbl)  [unwired: 1 in, 4 out]
            n114 = call "cluster2camera.vi"("Camera Device IN"=w369) -> ("Error OUT"=w372:errorcluster, "hCamera OUT"=w373:u32)  [unwired: 1 in]
            n115 = flat-sequence {
              tunnel: w373 -> [w377]
              tunnel: w372 -> [w376]
              tunnel: [w375] -> w367
              tunnel: [w374] -> w366
              tunnel: w365 -> [w393]
              tunnel: [w392] -> w371
              tunnel: [w391] -> w370
              tunnel: w367 -> [w390]
              tunnel: w366 -> [w389]
              tunnel: [w383] -> w364
              tunnel: w363 -> [w382]
              frame #0 {
                n116 = call "StartStopCamera.vi"("Error IN"=w376, "Camara ON?"=FALSE, "hCamera IN"=w377) -> ("Error OUT"=w374:errorcluster, "hCamera OUT"=w375:u32)  [unwired: 1 in]
              }
              frame #1 {
                w387 = T5 1 items=["FEATURE_FLAG_PRESENCE                 0x00000001", "FEATURE_FLAG_MANUAL                     0x00000002", "FEATURE_FLAG_AUTO                         0x00000004", "FEATURE_FLAG_ONEPUSH                   0x00000008", "FEATURE_FLAG_OFF                            0x00000010", "FEATURE_FLAG_DESC_SUPPORTED    0x00000020", "FEATURE_FLAG_READ_ONLY               0x00000040"] ("uFlags IN")
                w388 = T6 11 items=["FEATURE_BRIGHTNESS", "FEATURE_EXPOSURE", "FEATURE_SHARPNESS", "FEATURE_WHITE_BAL", "FEATURE_HUE", "FEATURE_SATURATION", "FEATURE_GAMMA", "FEATURE_SHUTTER", "FEATURE_GAIN", "FEATURE_IRIS", "FEATURE_FOCUS", "FEATURE_TEMPERATURE", "FEATURE_TRIGGER", "FEATURE_ZOOM", "FEATURE_PAN", "FEATURE_TILT", "FEATURE_OPT_FILTER", "FEATURE_GPIO", "FEATURE_FRAME_RATE", "FEATURE_ROI", "FEATURE_FLIP", "FEATURE_PIXEL_ADDRESSING", "FEATURE_PIXEL_FORMAT", "FEATURE_EXTENDED_SHUTTER", "FEATURE_AUTO_ROI", "FEATURE_LOOKUP_TABLE", "FEATURE_MEMORY_CHANNEL", "FEATURE_WHITE_SHADING", "FEATURE_ROTATE", "FEATURE_IMAGER_CLK_DIVISOR", "FEATURE_TRIG_WITH_CNTRLD_LIGHT", "FEATURE_MAX_PIXEL_SIZE"] ("uFeatureId IN")
                n117 = call <vilib>:"MEPU-CameraFeatures-SetFeature.vi"("hCamera IN"=w390, "uFeatureId IN"=w388, "uFlags IN"=w387, "pParms IN"=w382, "Error IN"=w389) -> ("hCamera OUT"=w386:u32, "Error OUT"=w381:errorcluster)  [unwired: 8 in, 1 out]
                n118 = call "showError.vi"("message"="Ocurrio un error con el Color Temperature", "Error IN"=w381) -> ("Error OUT"=w380:errorcluster)  [unwired: 3 in]
                n119 = call "getCameraParameters.vi"("Error IN"=w380, "hCamera IN"=w386) -> ("Error OUT"=w384:errorcluster, "Camera Parameters"=w383:T3, "hCamera OUT"=w385:u32)  [unwired: 1 in]
                n120 = call "StartStopCamera.vi"("Error IN"=w384, "Camara ON?"=w393, "hCamera IN"=w385) -> ("Error OUT"=w391:errorcluster, "hCamera OUT"=w392:u32)  [unwired: 1 in]
              }
            }
            n121 = To Double Precision Float(number=w361) -> (double precision float=w360:dbl)
            n122 = Build Array(w360) -> (w363:dbl[])
            n123 = call "camera2cluster.vi"("Error IN"=w370, "hCamera IN"=w371) -> ("Camera Device OUT"=w368:T1)  [unwired: 1 in]
          }
        }
      }
    }
  }
  "Camera Device OUT" <- w7
  n124 = property on="Camera Parameters" class="Clust (strict)"("Value"=w8) -> ()  [unwired: 2 in, 2 out]
